vi "array -- find closest element.vi"(8 "number":dbl, 11 "Array":dbl[](array[numeric])) -> (0 "value":dbl, 1 "index":i32)   [LabVIEW 2015]
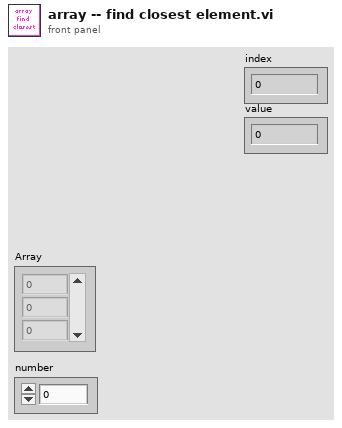
[diagram p1: front panel]
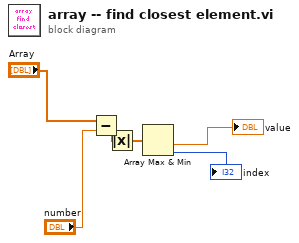
[diagram p0: block diagram]
diagram:
  n1 = Subtract(x="Array", y="number") -> (x-y=w6:dbl[])
  n2 = Absolute Value(x=w6) -> (abs(x)=w5:dbl[])
  n3 = Array Max & Min(array=w5) -> (min value=→"value":dbl, min index (indices)=→"index":i32)  [unwired: 2 out]
